vi "modulo.vi"(10 "Input":dbl) -> (2 "Modulo 3":bool)   [LabVIEW 2022 SP3]
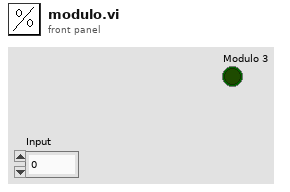
[diagram p1: front panel]
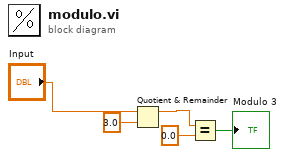
[diagram p0: block diagram]
diagram:
  n1 = Quotient & Remainder(x="Input", y=3.0) -> (x-y*floor(x/y)=w2:dbl)  [unwired: 1 out]
  n2 = Equal?(x=w2, y=0.0) -> (x = y?=→"Modulo 3":bool)
